vi "MAIN XY und Z gemeinsam Test.vi"() -> ()   [LabVIEW 2017]
uses:
  C:/Program Files (x86)/National Instruments/LabVIEW 2017/examples/Instrument IO/Serial/support/Serial - Settings.ctl
  <vilib>/Instr/_visa.llb/VISA Configure Serial Port (Instr).vi
panel:
  in  "XY_M_MotorOff":bool
  in  "XY_M_MotorOn":bool
  in  "XY_L_X":bool
  in  "XY_L_KonKreise":bool
  in  "XY_M_Center":bool
  in  "XY_L_Kreis_X":bool
  in  "XY_M_Relative":bool
  in  "XY_M_Move":bool
  in  "XY_M_Trigger":bool
  in  "Stopp 2":bool
  in  "X rel":i32
  in  "Y rel":i32
  in  "X":i32 min=0 max=15000
  in  "Y":i32 min=0 max=15000
  out "Antwort 2":string
  in  "VISA-Ressourcenname 2":refnum<visa-resource-name>="COM13"
  in  "Einstellungen des seriellen Ports 2":T1={"Baudrate"=19200, "Datenbits"=8, "Parität"=enum."None", "Stoppbits"=10, "Ablaufsteuerung"=0} {"Ablaufsteuerung" items=["Keine"=0, "XON/XOFF"=1, "RTS/CTS"=2, "DTR/DSR"=4]; "Stoppbits" items=["1,0"=10, "1,5"=15, "2,0"=20]; "Datenbits" min=5 max=8 step=1; "Baudrate" items=["75"=75, "110"=110, "134"=134, "150"=150, "300"=300, "600"=600, "1200"=1200, "1800"=1800, "2400"=2400, "4800"=4800, "7200"=7200, "9600"=9600, "14400"=14400, "19200"=19200, "28800"=28800, "38400"=38400, "56000"=56000, "57600"=57600, "115200"=115200, "128000"=128000, "230400"=230400]}
  in  "Z_M_Center":bool
  in  "Z_M_Fokus":bool
  in  "Z_M_Position":bool
  in  "Z_D_absWinkel":bool
  in  "Z_M_Trigger":bool
  in  "Stopp":bool
  in  "Pos (0 - 72000)":i32
  in  "Winkel (gon)":i32 min=0 max=15000
  out "Antwort":string
  in  "VISA-Ressourcenname":refnum<visa-resource-name>="COM13"
  in  "Einstellungen des seriellen Ports":T1={"Baudrate"=19200, "Datenbits"=8, "Parität"=enum."None", "Stoppbits"=10, "Ablaufsteuerung"=0} {"Ablaufsteuerung" items=["Keine"=0, "XON/XOFF"=1, "RTS/CTS"=2, "DTR/DSR"=4]; "Stoppbits" items=["1,0"=10, "1,5"=15, "2,0"=20]; "Datenbits" min=5 max=8 step=1; "Baudrate" items=["75"=75, "110"=110, "134"=134, "150"=150, "300"=300, "600"=600, "1200"=1200, "1800"=1800, "2400"=2400, "4800"=4800, "7200"=7200, "9600"=9600, "14400"=14400, "19200"=19200, "28800"=28800, "38400"=38400, "56000"=56000, "57600"=57600, "115200"=115200, "128000"=128000, "230400"=230400]}
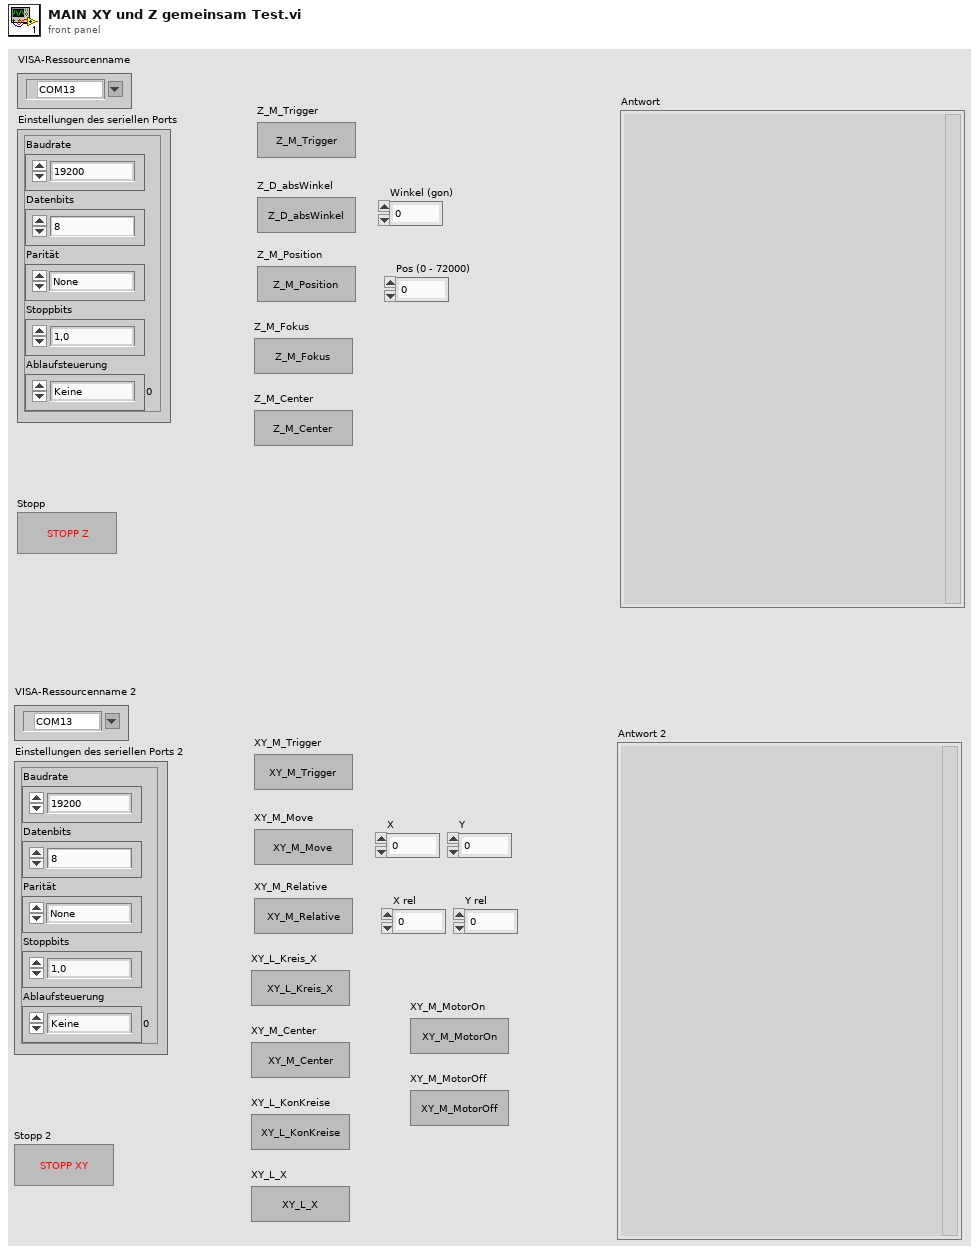
[diagram p1: front panel]
types:
  T1 = typedef "Serial - Settings.ctl" = cluster{"Baudrate":u32, "Datenbits":u16, "Parität":enum16{"None", "Odd", "Even", "Mark", "Space"}, "Stoppbits":u16, "Ablaufsteuerung":u16}
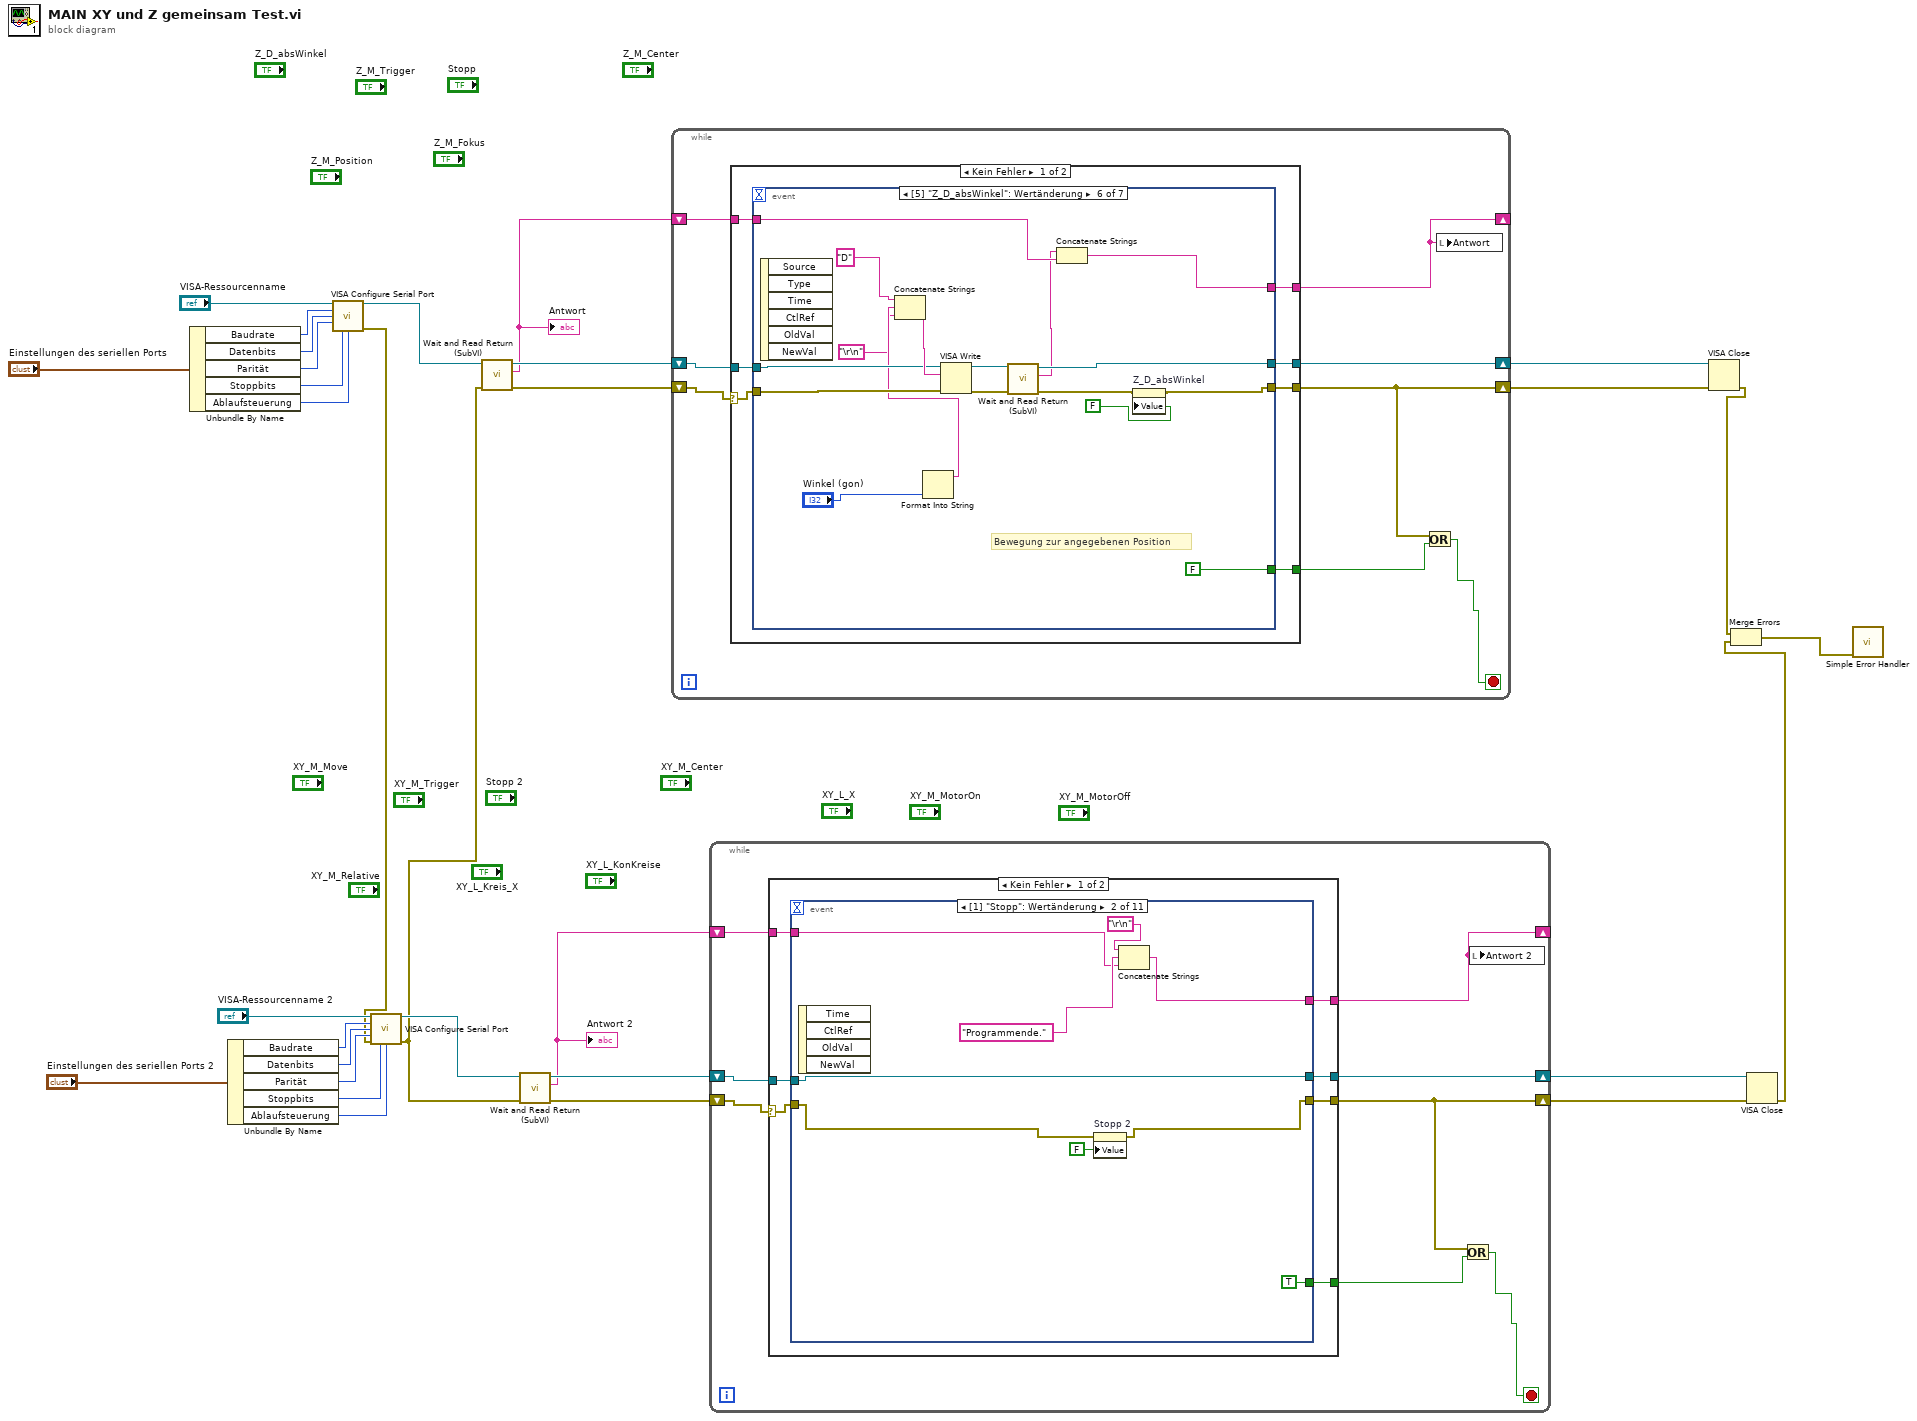
[diagram p0: block diagram]
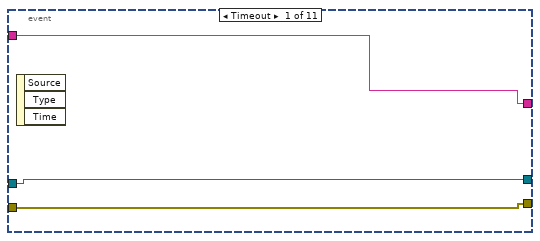
[diagram p2: hidden frame]
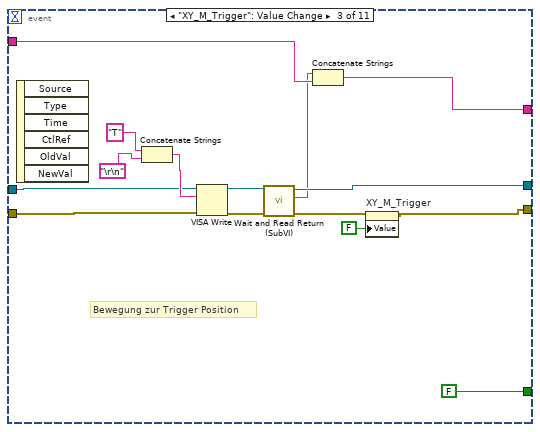
[diagram p3: hidden frame]
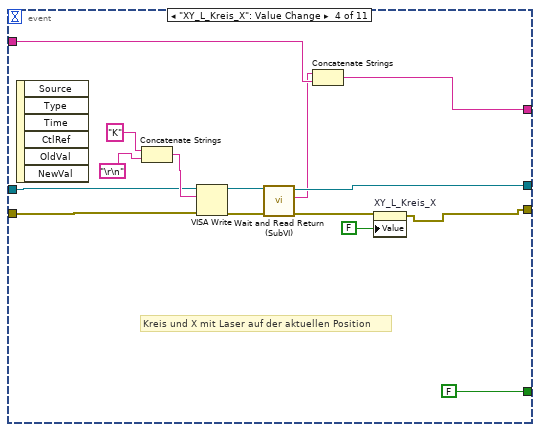
[diagram p4: hidden frame]
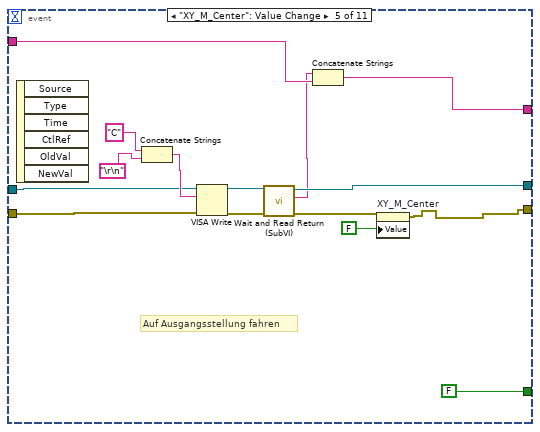
[diagram p5: hidden frame]
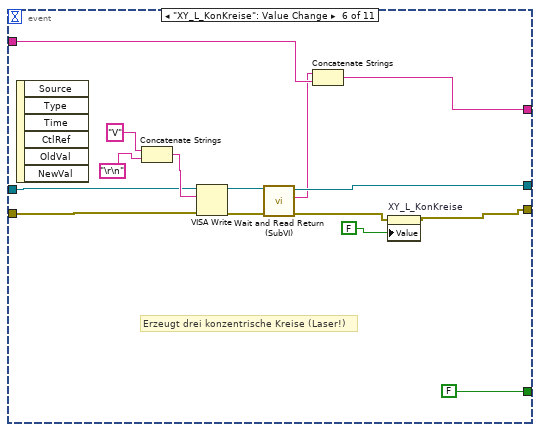
[diagram p6: hidden frame]
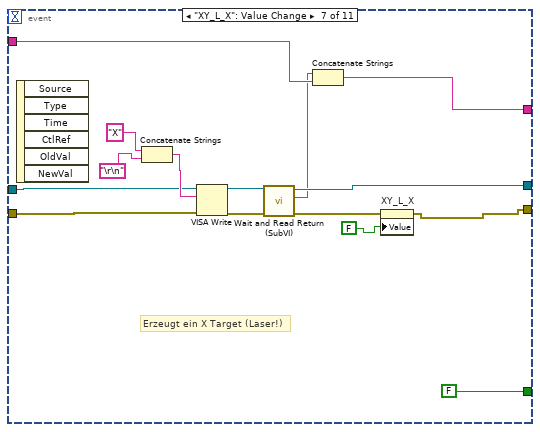
[diagram p7: hidden frame]
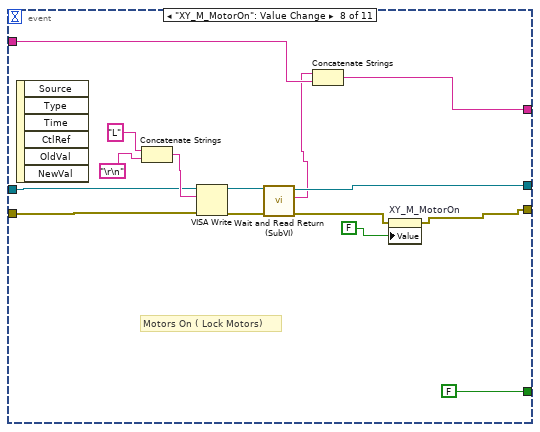
[diagram p8: hidden frame]
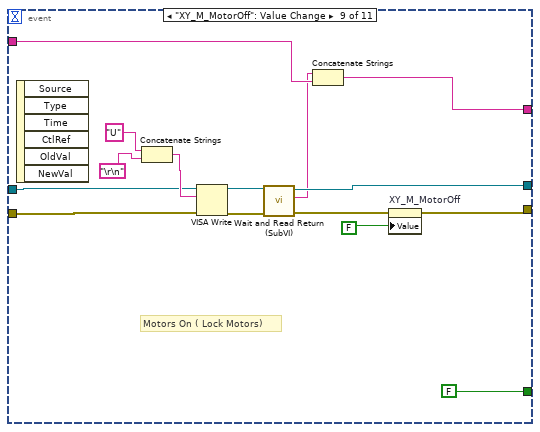
[diagram p9: hidden frame]
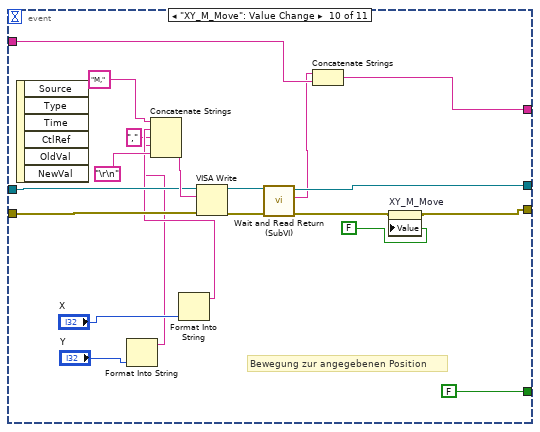
[diagram p10: hidden frame]
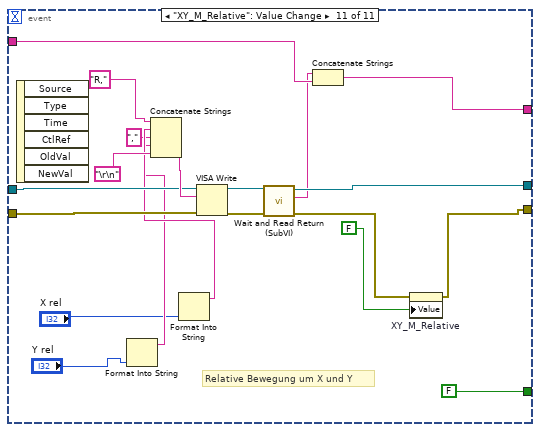
[diagram p11: hidden frame]
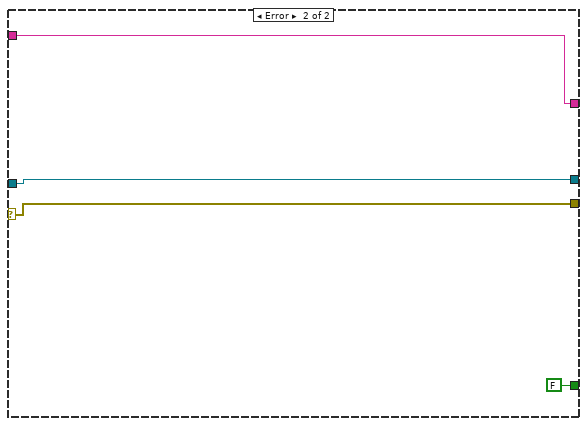
[diagram p12: hidden frame]
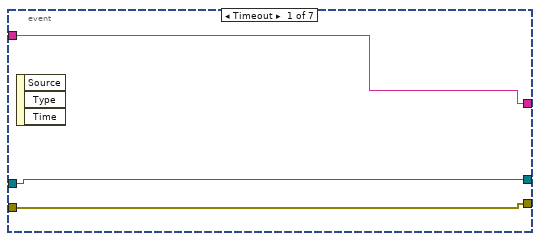
[diagram p13: hidden frame]
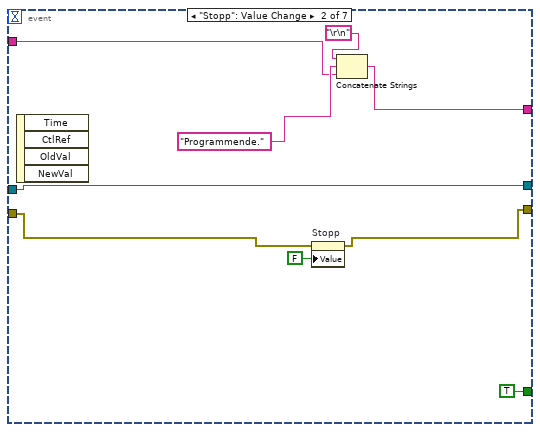
[diagram p14: hidden frame]
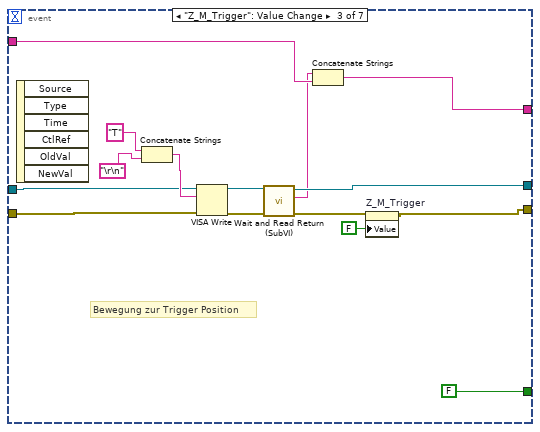
[diagram p15: hidden frame]
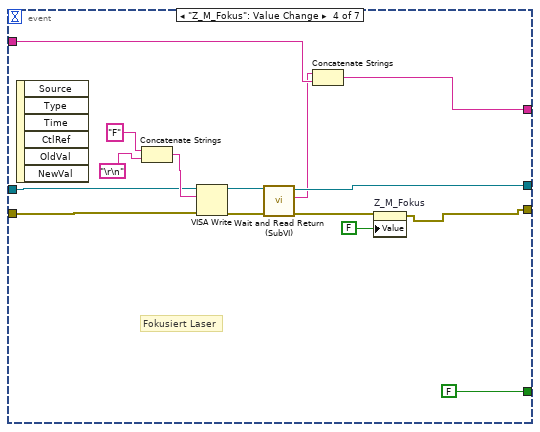
[diagram p16: hidden frame]
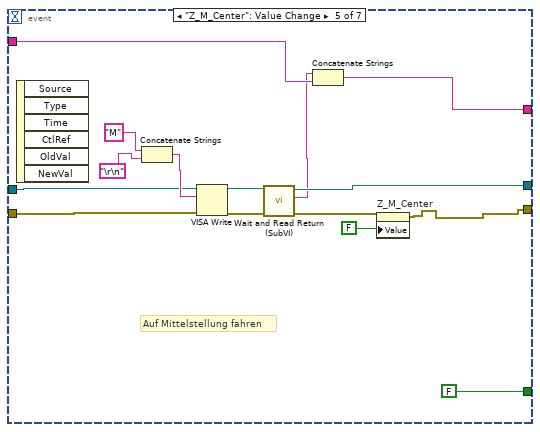
[diagram p17: hidden frame]
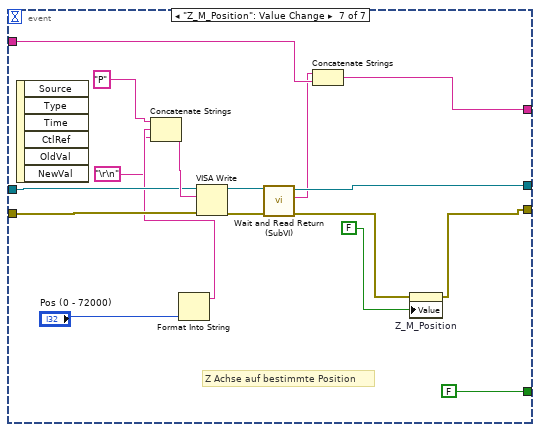
[diagram p18: hidden frame]
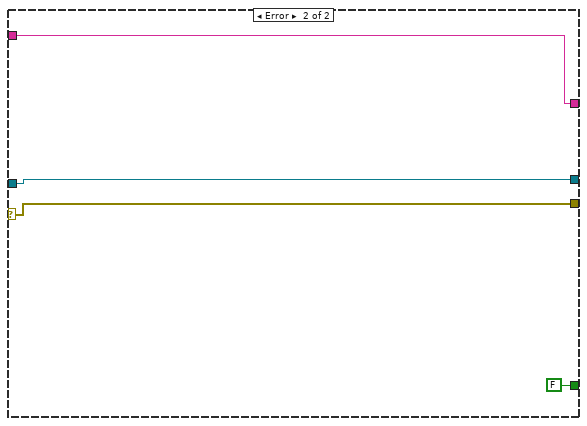
[diagram p19: hidden frame]
diagram:
  n1 = Unbundle By Name("Einstellungen des seriellen Ports") -> ("Baudrate"=w27:u32, "Datenbits"=w28:u16, "Parität"=w29:enum16{"None", "Odd", "Even", "Mark", "Space"}, "Stoppbits"=w30:u16, "Ablaufsteuerung"=w25:u16)
  n2 = Unbundle By Name("Einstellungen des seriellen Ports 2") -> ("Baudrate"=w14:u32, "Datenbits"=w15:u16, "Parität"=w16:enum16{"None", "Odd", "Even", "Mark", "Space"}, "Stoppbits"=w17:u16, "Ablaufsteuerung"=w12:u16)
  n3 = call-poly "VISA Configure Serial Port"("VISA resource name"="VISA-Ressourcenname", "baud rate (9600)"=w27, "data bits (8)"=w28, "parity (0:none)"=w29, "stop bits (10: 1 bit)"=w30, "flow control (0:none)"=w25) -> ("VISA resource name out"=w24:refnum<visa-resource-name>, "error out"=w5:errorcluster)  [unwired: 4 in, 4 out]
  n4 = call-poly "VISA Configure Serial Port"("VISA resource name"="VISA-Ressourcenname 2", "baud rate (9600)"=w14, "data bits (8)"=w15, "parity (0:none)"=w16, "error in (no error)"=w5, "stop bits (10: 1 bit)"=w17, "flow control (0:none)"=w12) -> ("VISA resource name out"=w11:refnum<visa-resource-name>, "error out"=w4:errorcluster)  [unwired: 3 in, 4 out]
  n5 = call "Wait and Read Return (SubVI).vi"("Fehler (Eingang, kein Fehler)"=w4, "VISA-Referenz (Eingang)"=w24) -> ("Fehler (Ausgang)"=w22:errorcluster, "Antwort"=w19:string, "VISA-Referenz (Ausgang)"=w23:refnum<visa-resource-name>)  [unwired: 7 in]
  "Antwort" <- w19
  n6 = call "Wait and Read Return (SubVI).vi"("Fehler (Eingang, kein Fehler)"=w4, "VISA-Referenz (Eingang)"=w11) -> ("Fehler (Ausgang)"=w9:errorcluster, "Antwort"=w6:string, "VISA-Referenz (Ausgang)"=w10:refnum<visa-resource-name>)  [unwired: 7 in]
  "Antwort 2" <- w6
  n7 = while {
    shift-right: [w38] -> w21
    shift-left: w23 -> [w39]
    shift-right: [w35] -> w20
    shift-left: w22 -> [w32]
    shift-right: [w36] -> _
    shift-left: w19 -> [w37]
    stop <- w33 stop-if-true
    n8 = case shown="Kein Fehler" w32 {
      selector: w32 -> [w40 w141]
      tunnel: w39 -> [w46 w140]
      tunnel: [w45 w140] -> w38
      tunnel: w37 -> [w44 w139]
      tunnel: [w43 w139] -> w36
      tunnel: [w42 w141] -> w35
      tunnel: [w41 FALSE] -> w34
      frame No Error {
        n9 = event shown="[5] \"Z_D_absWinkel\": Wertänderung" {
          selector: _ -> [_ _ _ _ _ _ _]
          dyn-events: _ -> [_ _ _ _ _ _ _]
          timeout: _ -> [_ _ _ _ _ _ _]
          tunnel: w46 -> [w49 w58 w68 w83 w98 w117 w134]
          tunnel: w40 -> [w48 w55 w67 w82 w97 w116 w133]
          tunnel: [w49 w58 w66 w81 w96 w115 w132] -> w45
          tunnel: [w48 w54 w61 w76 w91 w109 w125] -> w42
          tunnel: [w47 w56 w64 w79 w94 w113 w130] -> w43
          tunnel: [_ TRUE FALSE FALSE FALSE FALSE FALSE] -> w41
          tunnel: w44 -> [w47 w51 w60 w75 w90 w106 w123]
          event Timeout {
            n10 = event-data() -> ()  [unwired: 1 in, 3 out]
          }
          event "Stopp": Value Change {
            n11 = event-data() -> ()  [unwired: 1 in, 4 out]
            n12 = property on="Stopp" class="Bool. (strikt)"(error in=w55, "Value"=FALSE ("Stopp")) -> (error out=w54:errorcluster)  [unwired: 1 in, 1 out]
            n13 = Concatenate Strings("\r\n", "Programmende." ("String"), w51) -> (w56:string)
          }
          event "Z_M_Trigger": Value Change {
            # "Bewegung zur Trigger Position"
            n14 = event-data() -> ()  [unwired: 1 in, 6 out]
            n15 = Concatenate Strings("T" ("Schreibpuffer"), "\r\n") -> (w71:string)
            n16 = VISA Write(VISA resource name=w68, write buffer=w71, error in (no error)=w67) -> (VISA resource name out=w70:refnum<visa-resource-name>, error out=w69:errorcluster)  [unwired: 1 out]
            n17 = call "Wait and Read Return (SubVI).vi"("Fehler (Eingang, kein Fehler)"=w69, "VISA-Referenz (Eingang)"=w70) -> ("Fehler (Ausgang)"=w62:errorcluster, "Antwort"=w59:string, "VISA-Referenz (Ausgang)"=w66:refnum<visa-resource-name>)  [unwired: 7 in]
            n18 = Concatenate Strings(w59, w60) -> (w64:string)
            n19 = property on="Z_M_Trigger" class="Bool. (strikt)"(error in=w62, "Value"=FALSE ("XY_M_Trigger")) -> (error out=w61:errorcluster)  [unwired: 1 in, 1 out]
          }
          event "Z_M_Fokus": Value Change {
            # "Fokusiert Laser"
            n20 = event-data() -> ()  [unwired: 1 in, 6 out]
            n21 = Concatenate Strings("F" ("Schreibpuffer"), "\r\n") -> (w86:string)
            n22 = VISA Write(VISA resource name=w83, write buffer=w86, error in (no error)=w82) -> (VISA resource name out=w85:refnum<visa-resource-name>, error out=w84:errorcluster)  [unwired: 1 out]
            n23 = call "Wait and Read Return (SubVI).vi"("Fehler (Eingang, kein Fehler)"=w84, "VISA-Referenz (Eingang)"=w85) -> ("Fehler (Ausgang)"=w77:errorcluster, "Antwort"=w74:string, "VISA-Referenz (Ausgang)"=w81:refnum<visa-resource-name>)  [unwired: 7 in]
            n24 = Concatenate Strings(w74, w75) -> (w79:string)
            n25 = property on="Z_M_Fokus" class="Bool. (strikt)"(error in=w77, "Value"=FALSE ("XY_M_Trigger")) -> (error out=w76:errorcluster)  [unwired: 1 in, 1 out]
          }
          event "Z_M_Center": Value Change {
            # "Auf Mittelstellung fahren"
            n26 = event-data() -> ()  [unwired: 1 in, 6 out]
            n27 = Concatenate Strings("M" ("Schreibpuffer"), "\r\n") -> (w101:string)
            n28 = VISA Write(VISA resource name=w98, write buffer=w101, error in (no error)=w97) -> (VISA resource name out=w100:refnum<visa-resource-name>, error out=w99:errorcluster)  [unwired: 1 out]
            n29 = call "Wait and Read Return (SubVI).vi"("Fehler (Eingang, kein Fehler)"=w99, "VISA-Referenz (Eingang)"=w100) -> ("Fehler (Ausgang)"=w92:errorcluster, "Antwort"=w89:string, "VISA-Referenz (Ausgang)"=w96:refnum<visa-resource-name>)  [unwired: 7 in]
            n30 = Concatenate Strings(w89, w90) -> (w94:string)
            n31 = property on="Z_M_Center" class="Bool. (strikt)"(error in=w92, "Value"=FALSE ("XY_M_Trigger")) -> (error out=w91:errorcluster)  [unwired: 1 in, 1 out]
          }
          event "Z_D_absWinkel": Value Change {
            # "Bewegung zur angegebenen Position"
            n32 = event-data() -> ()  [unwired: 1 in, 6 out]
            n33 = Format Into String("Winkel (gon)") -> (resulting string=w110:string)  [unwired: 3 in, 1 out]
            n34 = Concatenate Strings("D" ("Schreibpuffer"), w110, "\r\n") -> (w120:string)
            n35 = VISA Write(VISA resource name=w117, write buffer=w120, error in (no error)=w116) -> (VISA resource name out=w119:refnum<visa-resource-name>, error out=w118:errorcluster)  [unwired: 1 out]
            n36 = call "Wait and Read Return (SubVI).vi"("Fehler (Eingang, kein Fehler)"=w118, "VISA-Referenz (Eingang)"=w119) -> ("Fehler (Ausgang)"=w108:errorcluster, "Antwort"=w105:string, "VISA-Referenz (Ausgang)"=w115:refnum<visa-resource-name>)  [unwired: 7 in]
            n37 = Concatenate Strings(w105, w106) -> (w113:string)
            n38 = property on="Z_D_absWinkel" class="Bool. (strikt)"(error in=w108, "Value"=FALSE ("XY_M_Trigger")) -> (error out=w109:errorcluster)  [unwired: 1 in, 1 out]
          }
          event "Z_M_Position": Value Change {
            # "Z Achse auf bestimmte Position"
            n39 = event-data() -> ()  [unwired: 1 in, 6 out]
            n40 = Format Into String("Pos (0 - 72000)") -> (resulting string=w128:string)  [unwired: 3 in, 1 out]
            n41 = Concatenate Strings("P" ("Schreibpuffer"), w128, "\r\n") -> (w137:string)
            n42 = VISA Write(VISA resource name=w134, write buffer=w137, error in (no error)=w133) -> (VISA resource name out=w136:refnum<visa-resource-name>, error out=w135:errorcluster)  [unwired: 1 out]
            n43 = call "Wait and Read Return (SubVI).vi"("Fehler (Eingang, kein Fehler)"=w135, "VISA-Referenz (Eingang)"=w136) -> ("Fehler (Ausgang)"=w126:errorcluster, "Antwort"=w122:string, "VISA-Referenz (Ausgang)"=w132:refnum<visa-resource-name>)  [unwired: 7 in]
            n44 = Concatenate Strings(w122, w123) -> (w130:string)
            n45 = property on="Z_M_Position" class="Bool. (strikt)"(error in=w126, "Value"=FALSE ("XY_M_Trigger")) -> (error out=w125:errorcluster)  [unwired: 1 in, 1 out]
          }
        }
      }
      frame Error {
      }
    }
    n46 = Or(x=w35, y=w34) -> (x .or. y?=w33:bool)
    n47 = local write "Antwort"(w36) -> ()
  }
  n48 = while {
    shift-right: [w148] -> w8
    shift-left: w10 -> [w149]
    shift-right: [w145] -> w7
    shift-left: w9 -> [w142]
    shift-right: [w146] -> _
    shift-left: w6 -> [w147]
    stop <- w143 stop-if-true
    n49 = case shown="Kein Fehler" w142 {
      selector: w142 -> [w150 w317]
      tunnel: w149 -> [w156 w316]
      tunnel: [w155 w316] -> w148
      tunnel: w147 -> [w154 w315]
      tunnel: [w153 w315] -> w146
      tunnel: [w152 w317] -> w145
      tunnel: [w151 FALSE] -> w144
      frame No Error {
        n50 = event shown="[1] \"Stopp\": Wertänderung" {
          selector: _ -> [_ _ _ _ _ _ _ _ _ _ _]
          dyn-events: _ -> [_ _ _ _ _ _ _ _ _ _ _]
          timeout: _ -> [_ _ _ _ _ _ _ _ _ _ _]
          tunnel: w156 -> [w159 w168 w178 w193 w208 w223 w238 w253 w268 w289 w309]
          tunnel: w150 -> [w158 w165 w177 w192 w207 w222 w237 w252 w267 w288 w308]
          tunnel: [w159 w168 w176 w191 w206 w221 w236 w251 w266 w287 w307] -> w155
          tunnel: [w158 w164 w171 w186 w201 w216 w231 w246 w261 w278 w298] -> w152
          tunnel: [w157 w166 w174 w189 w204 w219 w234 w249 w264 w285 w305] -> w153
          tunnel: [_ TRUE FALSE FALSE FALSE FALSE FALSE FALSE FALSE FALSE FALSE] -> w151
          tunnel: w154 -> [w157 w161 w170 w185 w200 w215 w230 w245 w260 w275 w295]
          event Timeout {
            n51 = event-data() -> ()  [unwired: 1 in, 3 out]
          }
          event "Stopp 2": Value Change {
            n52 = event-data() -> ()  [unwired: 1 in, 4 out]
            n53 = property on="Stopp 2" class="Bool. (strikt)"(error in=w165, "Value"=FALSE ("Stopp")) -> (error out=w164:errorcluster)  [unwired: 1 in, 1 out]
            n54 = Concatenate Strings("\r\n", "Programmende." ("String"), w161) -> (w166:string)
          }
          event "XY_M_Trigger": Value Change {
            # "Bewegung zur Trigger Position"
            n55 = event-data() -> ()  [unwired: 1 in, 6 out]
            n56 = Concatenate Strings("T" ("Schreibpuffer"), "\r\n") -> (w181:string)
            n57 = VISA Write(VISA resource name=w178, write buffer=w181, error in (no error)=w177) -> (VISA resource name out=w180:refnum<visa-resource-name>, error out=w179:errorcluster)  [unwired: 1 out]
            n58 = call "Wait and Read Return (SubVI).vi"("Fehler (Eingang, kein Fehler)"=w179, "VISA-Referenz (Eingang)"=w180) -> ("Fehler (Ausgang)"=w172:errorcluster, "Antwort"=w169:string, "VISA-Referenz (Ausgang)"=w176:refnum<visa-resource-name>)  [unwired: 7 in]
            n59 = Concatenate Strings(w169, w170) -> (w174:string)
            n60 = property on="XY_M_Trigger" class="Bool. (strikt)"(error in=w172, "Value"=FALSE ("XY_M_Trigger")) -> (error out=w171:errorcluster)  [unwired: 1 in, 1 out]
          }
          event "XY_L_Kreis_X": Value Change {
            # "Kreis und X mit Laser auf der aktuellen Position"
            n61 = event-data() -> ()  [unwired: 1 in, 6 out]
            n62 = Concatenate Strings("K" ("Schreibpuffer"), "\r\n") -> (w196:string)
            n63 = VISA Write(VISA resource name=w193, write buffer=w196, error in (no error)=w192) -> (VISA resource name out=w195:refnum<visa-resource-name>, error out=w194:errorcluster)  [unwired: 1 out]
            n64 = call "Wait and Read Return (SubVI).vi"("Fehler (Eingang, kein Fehler)"=w194, "VISA-Referenz (Eingang)"=w195) -> ("Fehler (Ausgang)"=w187:errorcluster, "Antwort"=w184:string, "VISA-Referenz (Ausgang)"=w191:refnum<visa-resource-name>)  [unwired: 7 in]
            n65 = Concatenate Strings(w184, w185) -> (w189:string)
            n66 = property on="XY_L_Kreis_X" class="Bool. (strikt)"(error in=w187, "Value"=FALSE ("XY_M_Trigger")) -> (error out=w186:errorcluster)  [unwired: 1 in, 1 out]
          }
          event "XY_M_Center": Value Change {
            # "Auf Ausgangsstellung fahren"
            n67 = event-data() -> ()  [unwired: 1 in, 6 out]
            n68 = Concatenate Strings("C" ("Schreibpuffer"), "\r\n") -> (w211:string)
            n69 = VISA Write(VISA resource name=w208, write buffer=w211, error in (no error)=w207) -> (VISA resource name out=w210:refnum<visa-resource-name>, error out=w209:errorcluster)  [unwired: 1 out]
            n70 = call "Wait and Read Return (SubVI).vi"("Fehler (Eingang, kein Fehler)"=w209, "VISA-Referenz (Eingang)"=w210) -> ("Fehler (Ausgang)"=w202:errorcluster, "Antwort"=w199:string, "VISA-Referenz (Ausgang)"=w206:refnum<visa-resource-name>)  [unwired: 7 in]
            n71 = Concatenate Strings(w199, w200) -> (w204:string)
            n72 = property on="XY_M_Center" class="Bool. (strikt)"(error in=w202, "Value"=FALSE ("XY_M_Trigger")) -> (error out=w201:errorcluster)  [unwired: 1 in, 1 out]
          }
          event "XY_L_KonKreise": Value Change {
            # "Erzeugt drei konzentrische Kreise (Laser!)"
            n73 = event-data() -> ()  [unwired: 1 in, 6 out]
            n74 = Concatenate Strings("V" ("Schreibpuffer"), "\r\n") -> (w226:string)
            n75 = VISA Write(VISA resource name=w223, write buffer=w226, error in (no error)=w222) -> (VISA resource name out=w225:refnum<visa-resource-name>, error out=w224:errorcluster)  [unwired: 1 out]
            n76 = call "Wait and Read Return (SubVI).vi"("Fehler (Eingang, kein Fehler)"=w224, "VISA-Referenz (Eingang)"=w225) -> ("Fehler (Ausgang)"=w217:errorcluster, "Antwort"=w214:string, "VISA-Referenz (Ausgang)"=w221:refnum<visa-resource-name>)  [unwired: 7 in]
            n77 = Concatenate Strings(w214, w215) -> (w219:string)
            n78 = property on="XY_L_KonKreise" class="Bool. (strikt)"(error in=w217, "Value"=FALSE ("XY_M_Trigger")) -> (error out=w216:errorcluster)  [unwired: 1 in, 1 out]
          }
          event "XY_L_X": Value Change {
            # "Erzeugt ein X Target (Laser!)"
            n79 = event-data() -> ()  [unwired: 1 in, 6 out]
            n80 = Concatenate Strings("X" ("Schreibpuffer"), "\r\n") -> (w241:string)
            n81 = VISA Write(VISA resource name=w238, write buffer=w241, error in (no error)=w237) -> (VISA resource name out=w240:refnum<visa-resource-name>, error out=w239:errorcluster)  [unwired: 1 out]
            n82 = call "Wait and Read Return (SubVI).vi"("Fehler (Eingang, kein Fehler)"=w239, "VISA-Referenz (Eingang)"=w240) -> ("Fehler (Ausgang)"=w232:errorcluster, "Antwort"=w229:string, "VISA-Referenz (Ausgang)"=w236:refnum<visa-resource-name>)  [unwired: 7 in]
            n83 = Concatenate Strings(w229, w230) -> (w234:string)
            n84 = property on="XY_L_X" class="Bool. (strikt)"(error in=w232, "Value"=FALSE ("XY_M_Trigger")) -> (error out=w231:errorcluster)  [unwired: 1 in, 1 out]
          }
          event "XY_M_MotorOn": Value Change {
            # "Motors On ( Lock Motors)"
            n85 = event-data() -> ()  [unwired: 1 in, 6 out]
            n86 = Concatenate Strings("L" ("Schreibpuffer"), "\r\n") -> (w256:string)
            n87 = VISA Write(VISA resource name=w253, write buffer=w256, error in (no error)=w252) -> (VISA resource name out=w255:refnum<visa-resource-name>, error out=w254:errorcluster)  [unwired: 1 out]
            n88 = call "Wait and Read Return (SubVI).vi"("Fehler (Eingang, kein Fehler)"=w254, "VISA-Referenz (Eingang)"=w255) -> ("Fehler (Ausgang)"=w247:errorcluster, "Antwort"=w244:string, "VISA-Referenz (Ausgang)"=w251:refnum<visa-resource-name>)  [unwired: 7 in]
            n89 = Concatenate Strings(w244, w245) -> (w249:string)
            n90 = property on="XY_M_MotorOn" class="Bool. (strikt)"(error in=w247, "Value"=FALSE ("XY_M_Trigger")) -> (error out=w246:errorcluster)  [unwired: 1 in, 1 out]
          }
          event "XY_M_MotorOff": Value Change {
            # "Motors On ( Lock Motors)"
            n91 = event-data() -> ()  [unwired: 1 in, 6 out]
            n92 = Concatenate Strings("U" ("Schreibpuffer"), "\r\n") -> (w271:string)
            n93 = VISA Write(VISA resource name=w268, write buffer=w271, error in (no error)=w267) -> (VISA resource name out=w270:refnum<visa-resource-name>, error out=w269:errorcluster)  [unwired: 1 out]
            n94 = call "Wait and Read Return (SubVI).vi"("Fehler (Eingang, kein Fehler)"=w269, "VISA-Referenz (Eingang)"=w270) -> ("Fehler (Ausgang)"=w262:errorcluster, "Antwort"=w259:string, "VISA-Referenz (Ausgang)"=w266:refnum<visa-resource-name>)  [unwired: 7 in]
            n95 = Concatenate Strings(w259, w260) -> (w264:string)
            n96 = property on="XY_M_MotorOff" class="Bool. (strikt)"(error in=w262, "Value"=FALSE ("XY_M_Trigger")) -> (error out=w261:errorcluster)  [unwired: 1 in, 1 out]
          }
          event "XY_M_Move": Value Change {
            # "Bewegung zur angegebenen Position"
            n97 = event-data() -> ()  [unwired: 1 in, 6 out]
            n98 = Format Into String("Y") -> (resulting string=w280:string)  [unwired: 3 in, 1 out]
            n99 = Format Into String("X") -> (resulting string=w281:string)  [unwired: 3 in, 1 out]
            n100 = Concatenate Strings("M," ("Schreibpuffer"), w281, "," ("String"), w280, "\r\n") -> (w292:string)
            n101 = VISA Write(VISA resource name=w289, write buffer=w292, error in (no error)=w288) -> (VISA resource name out=w291:refnum<visa-resource-name>, error out=w290:errorcluster)  [unwired: 1 out]
            n102 = call "Wait and Read Return (SubVI).vi"("Fehler (Eingang, kein Fehler)"=w290, "VISA-Referenz (Eingang)"=w291) -> ("Fehler (Ausgang)"=w277:errorcluster, "Antwort"=w274:string, "VISA-Referenz (Ausgang)"=w287:refnum<visa-resource-name>)  [unwired: 7 in]
            n103 = Concatenate Strings(w274, w275) -> (w285:string)
            n104 = property on="XY_M_Move" class="Bool. (strikt)"(error in=w277, "Value"=FALSE ("XY_M_Trigger")) -> (error out=w278:errorcluster)  [unwired: 1 in, 1 out]
          }
          event "XY_M_Relative": Value Change {
            # "Relative Bewegung um X und Y"
            n105 = event-data() -> ()  [unwired: 1 in, 6 out]
            n106 = Format Into String("Y rel") -> (resulting string=w302:string)  [unwired: 3 in, 1 out]
            n107 = Format Into String("X rel") -> (resulting string=w303:string)  [unwired: 3 in, 1 out]
            n108 = Concatenate Strings("R," ("Schreibpuffer"), w303, "," ("String"), w302, "\r\n") -> (w312:string)
            n109 = VISA Write(VISA resource name=w309, write buffer=w312, error in (no error)=w308) -> (VISA resource name out=w311:refnum<visa-resource-name>, error out=w310:errorcluster)  [unwired: 1 out]
            n110 = call "Wait and Read Return (SubVI).vi"("Fehler (Eingang, kein Fehler)"=w310, "VISA-Referenz (Eingang)"=w311) -> ("Fehler (Ausgang)"=w299:errorcluster, "Antwort"=w294:string, "VISA-Referenz (Ausgang)"=w307:refnum<visa-resource-name>)  [unwired: 7 in]
            n111 = Concatenate Strings(w294, w295) -> (w305:string)
            n112 = property on="XY_M_Relative" class="Bool. (strikt)"(error in=w299, "Value"=FALSE ("XY_M_Trigger")) -> (error out=w298:errorcluster)  [unwired: 1 in, 1 out]
          }
        }
      }
      frame Error {
      }
    }
    n113 = Or(x=w145, y=w144) -> (x .or. y?=w143:bool)
    n114 = local write "Antwort 2"(w146) -> ()
  }
  n115 = VISA Close(VISA resource name=w21, error in (no error)=w20) -> (error out=w3:errorcluster)
  n116 = VISA Close(VISA resource name=w8, error in (no error)=w7) -> (error out=w2:errorcluster)
  n117 = Merge Errors(w3, w2) -> (w1:errorcluster)
  n118 = call <vilib>:"Simple Error Handler.vi"("error in (no error)"=w1) -> ()  [unwired: 4 in, 5 out]
